vi "PathSearch.vi"(0 "Path":dbl[][](array[numeric]), 5 "Reint":bool, 9 "Robot X (in)":dbl, 11 "Robot Y (in)":dbl, 12 "Search Window (s)":dbl=2.0, 13 "Look-Ahead Time (s)":dbl=0.25) -> (1 "Distance from Start (in)":dbl, 3 "Distance from End (in)":dbl, 4 "Feed Back Distance Error (in)":dbl, 6 "Feed Back Pointing Angle (deg)":dbl, 8 "Feed Forward Pointing Angle (deg)":dbl, 10 "Feed Forward Velocity (in/s)":dbl, 15 "Robot Heading Goal (deg)":dbl)   [LabVIEW 2019]
doc: "This VI takes as input the robots current pose and the loaded autonomous path. The algorithm then efficiently searches the path and identifies the nearest point and the pursuit point. The the feed-forward heading, pointing direction, and velocity are output along with the error distance and and pointing direction required to return to the path. The distance along the path is also output. The Search Window can be specified in seconds - longer search windows are more robust to recovering from large deviations from the path but may cause the robot to \"jump\" ahead when following tight loops or turns. The Look-Ahead Time specifies the furthest ahead the pursuit point can be."
panel:
  out "Look-Ahead Point":i32
  out "Closest Point":i32
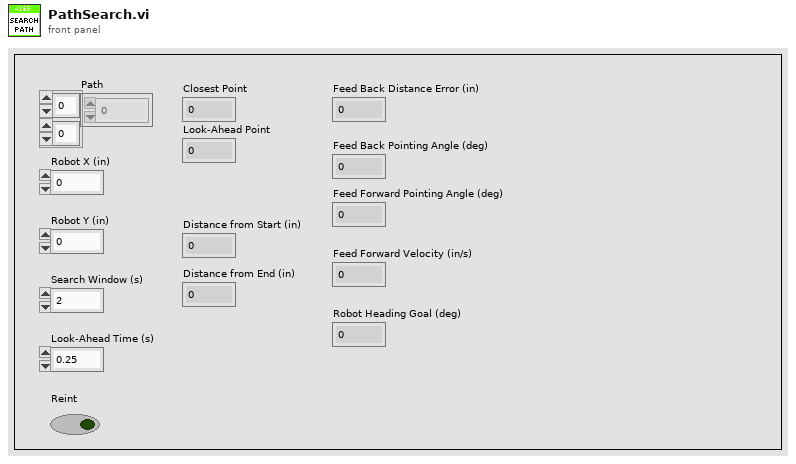
[diagram p1: front panel]
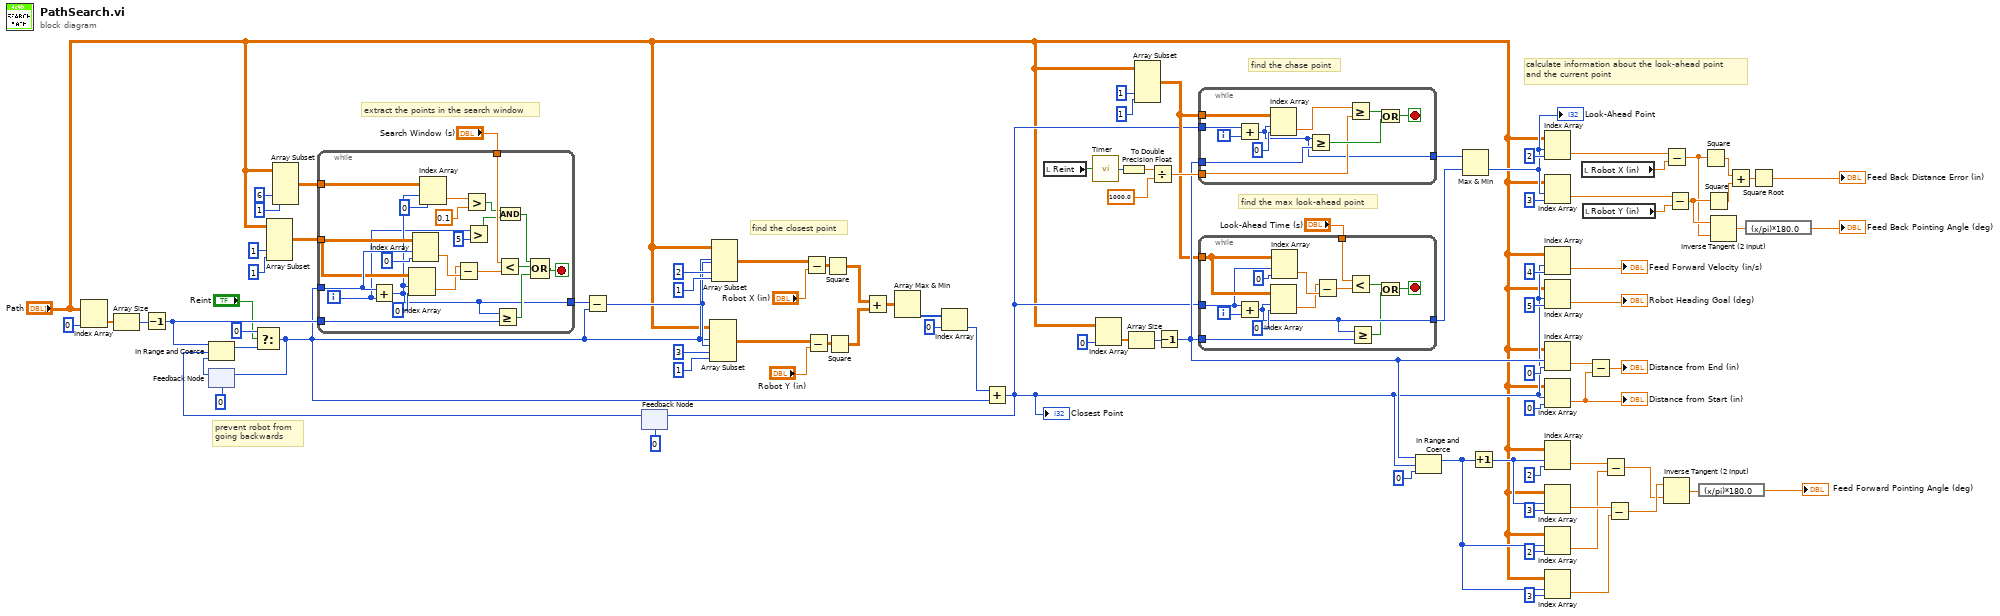
[diagram p0: block diagram]
diagram:
  # "find the chase point"
  # "find the max look-ahead point"
  # "calculate information about the look-ahead point\nand the current point"
  # "prevent robot from \ngoing backwards"
  # "find the closest point"
  # "extract the points in the search window"
  n1 = Index Array(array="Path", index (col)=0 ("disabled index (col)")) -> (element=w55:dbl[])  [unwired: 1 in]
  n2 = Array Size(array=w55) -> (size(s)=w56:i32)
  n3 = Decrement(x=w56) -> (x-1=w52:i32)
  n4 = feedback #1(0) -> (w53:i32)
  n5 = Array Subset(array="Path", index (col)=1 ("index"), length (col)=1 ("length")) -> (w76:dbl[][])  [unwired: 2 in]
  n6 = Array Subset(array="Path", index (col)=6 ("index"), length (col)=1 ("length")) -> (w1:dbl[][])  [unwired: 2 in]
  n7 = feedback #2(0) -> (w51:i32)
  n8 = In Range and Coerce(upper limit=w52, x=w51, lower limit=w53) -> (coerced(x)=w34:i32)  [unwired: 1 out]
  n9 = Select(t=0, s="Reint", f=w34) -> (s? t:f=w33:i32)
  n10 = feedback-in #1(w33) -> ()
  n11 = while {
    tunnel: w33 -> [w114]
    tunnel: w76 -> [w104]
    tunnel: "Search Window (s)" -> [w109]
    tunnel: [w99] -> w74
    tunnel: w52 -> [w105]
    tunnel: w1 -> [w103]
    i -> [w96]
    stop <- w107 stop-if-true
    # "Search window"
    n12 = Add(x=w114, y=w96) -> (x+y=w99:i32)
    n13 = Index Array(array=w104, index (row)=w99, index (col)=0 ("disabled index (col)")) -> (element=w111:dbl)
    n14 = Index Array(array=w104, index (row)=w114, index (col)=0 ("disabled index (col)")) -> (element=w112:dbl)
    n15 = Index Array(array=w103, index (row)=w99, index (col)=0 ("disabled index (col)")) -> (element=w102:dbl)
    n16 = Subtract(x=w111, y=w112) -> (x-y=w110:dbl)
    n17 = Greater?(x=w102, y=0.1) -> (0:w98:bool)
    n18 = Greater?(x=w96, y=5) -> (0:w97:bool)
    n19 = Greater Or Equal?(x=w99, y=w105) -> (x >= y?=w106:bool)
    n20 = Less?(x=w109, y=w110) -> (x < y?=w108:bool)
    n21 = And(x=w98, y=w97) -> (x .and. y?=w94:bool)
    n22 = Compound Arithmetic op=OR(w94, w108, w106) -> (w107:bool)
  }
  n23 = Subtract(x=w74, y=w33) -> (x-y=w73:i32)
  n24 = Array Subset(array="Path", index (row)=w33, length (row)=w73, index (col)=3 ("index"), length (col)=1 ("length")) -> (w85:dbl[][])
  n25 = Array Subset(array="Path", index (row)=w33, length (row)=w73, index (col)=2 ("index"), length (col)=1 ("length")) -> (w91:dbl[][])
  n26 = Subtract(x=w91, y="Robot X (in)") -> (x-y=w90:dbl[][])
  n27 = Subtract(x=w85, y="Robot Y (in)") -> (x-y=w86:dbl[][])
  n28 = Square(x=w90) -> (x^2=w83:dbl[][])
  n29 = Square(x=w86) -> (x^2=w82:dbl[][])
  n30 = Add(x=w83, y=w82) -> (x+y=w81:dbl[][])
  n31 = Array Max & Min(array=w81) -> (min index (indices)=w80:i32[])  [unwired: 3 out]
  n32 = Index Array(array=w80, index=0) -> (element=w72:i32)
  n33 = Add(x=w72, y=w33) -> (x+y=w5:i32)
  "Closest Point" <- w5
  n34 = feedback-in #2(w5) -> ()
  n35 = local read "Reint"() -> (w15:bool)
  n36 = call "Timer.vi"("Reset Timer"=w15) -> ("Time (ms)"=w14:u32)
  n37 = Index Array(array="Path", index (col)=0 ("disabled index (col)")) -> (element=w46:dbl[])  [unwired: 1 in]
  n38 = To Double Precision Float(number=w14) -> (double precision float=w12:dbl)
  n39 = Array Size(array=w46) -> (size(s)=w40:i32)
  n40 = Array Subset(array="Path", index (col)=1 ("index"), length (col)=1 ("length")) -> (w9:dbl[][])  [unwired: 2 in]
  n41 = Divide(x=w12, y=1000.0) -> (x/y=w11:dbl)
  n42 = Decrement(x=w40) -> (x-1=w10:i32)
  n43 = while {
    tunnel: w5 -> [w123]
    tunnel: w9 -> [w124]
    tunnel: w11 -> [w117]
    tunnel: w10 -> [w119]
    tunnel: [w116] -> w8
    i -> [w126]
    stop <- w121 stop-if-true
    # "Search window"
    n44 = Add(x=w123, y=w126) -> (x+y=w116:i32)
    n45 = Index Array(array=w124, index (row)=w116, index (col)=0 ("disabled index (col)")) -> (element=w118:dbl)
    n46 = Greater Or Equal?(x=w116, y=w119) -> (x >= y?=w120:bool)
    n47 = Greater Or Equal?(x=w118, y=w117) -> (x >= y?=w122:bool)
    n48 = Or(x=w122, y=w120) -> (x .or. y?=w121:bool)
  }
  n49 = while {
    tunnel: w5 -> [w137]
    tunnel: w9 -> [w138]
    tunnel: "Look-Ahead Time (s)" -> [w132]
    tunnel: [w131] -> w7
    tunnel: w10 -> [w127]
    i -> [w140]
    stop <- w129 stop-if-true
    # "Search window"
    n50 = Add(x=w137, y=w140) -> (x+y=w131:i32)
    n51 = Index Array(array=w138, index (row)=w131, index (col)=0 ("disabled index (col)")) -> (element=w134:dbl)
    n52 = Index Array(array=w138, index (row)=w137, index (col)=0 ("disabled index (col)")) -> (element=w135:dbl)
    n53 = Subtract(x=w134, y=w135) -> (x-y=w133:dbl)
    n54 = Less?(x=w132, y=w133) -> (x < y?=w130:bool)
    n55 = Greater Or Equal?(x=w131, y=w127) -> (x >= y?=w128:bool)
    n56 = Or(x=w130, y=w128) -> (x .or. y?=w129:bool)
  }
  n57 = In Range and Coerce(upper limit=w10, x=w5, lower limit=0) -> (coerced(x)=w18:i32)  [unwired: 1 out]
  n58 = Max & Min(x=w8, y=w7) -> (min(x,y)=w6:i32)  [unwired: 1 out]
  "Look-Ahead Point" <- w6
  n59 = Increment(x=w18) -> (x+1=w27:i32)
  n60 = Index Array(array="Path", index (row)=w6, index (col)=2 ("disabled index (col)")) -> (element=w69:dbl)
  n61 = Index Array(array="Path", index (row)=w6, index (col)=3 ("disabled index (col)")) -> (element=w67:dbl)
  n62 = Index Array(array="Path", index (row)=w5, index (col)=4 ("disabled index (col)")) -> (element=→"Feed Forward Velocity (in/s)":dbl)
  n63 = Index Array(array="Path", index (row)=w5, index (col)=5 ("disabled index (col)")) -> (element=→"Robot Heading Goal (deg)":dbl)
  n64 = Index Array(array="Path", index (row)=w10, index (col)=0 ("disabled index (row)")) -> (element=w37:dbl)
  n65 = Index Array(array="Path", index (row)=w5, index (col)=0 ("disabled index (col)")) -> (element=w35:dbl)
  "Distance from Start (in)" <- w35
  n66 = Index Array(array="Path", index (row)=w27, index (col)=2 ("disabled index (col)")) -> (element=w25:dbl)
  n67 = Index Array(array="Path", index (row)=w27, index (col)=3) -> (element=w26:dbl)
  n68 = Index Array(array="Path", index (row)=w18, index (col)=2) -> (element=w22:dbl)
  n69 = Index Array(array="Path", index (row)=w18, index (col)=3) -> (element=w21:dbl)
  n70 = local read "Robot X (in)"() -> (w68:dbl)
  n71 = local read "Robot Y (in)"() -> (w66:dbl)
  n72 = Subtract(x=w37, y=w35) -> (x-y=→"Distance from End (in)":dbl)
  n73 = Subtract(x=w25, y=w22) -> (x-y=w20:dbl)
  n74 = Subtract(x=w26, y=w21) -> (x-y=w29:dbl)
  n75 = Subtract(x=w69, y=w68) -> (x-y=w60:dbl)
  n76 = Inverse Tangent (2 Input)(1:w20, 2:w29) -> (0:w17:dbl)
  n77 = Subtract(x=w67, y=w66) -> (x-y=w61:dbl)
  n78 = expression code="(x/pi)*180.0"(w17) -> (→"Feed Forward Pointing Angle (deg)":dbl)
  n79 = Square(x=w60) -> (x^2=w64:dbl)
  n80 = Square(x=w61) -> (x^2=w65:dbl)
  n81 = Inverse Tangent (2 Input)(1:w60, 2:w61) -> (0:w59:dbl)
  n82 = Add(x=w64, y=w65) -> (x+y=w63:dbl)
  n83 = expression code="(x/pi)*180.0"(w59) -> (→"Feed Back Pointing Angle (deg)":dbl)
  n84 = Square Root(x=w63) -> (sqrt(x)=→"Feed Back Distance Error (in)":dbl)
